vi "Encoder Angles.vi"(8 "Calibration Angle":dbl, 9 "Bottom Voltage":dbl, 10 "Top Voltage":dbl, 11 "AIDeviceRef Encoder":T1) -> (3 "Encoder Angle":dbl)   [LabVIEW 2013]
uses:
  <vilib>/Rock Robotics/WPI/AnalogChannel/WPI_AnalogChannelDevRef.ctl
  <vilib>/Rock Robotics/SystemInterfaces/Typedef/FPGA_TypedefAnalogModule.ctl
  <vilib>/Rock Robotics/SystemInterfaces/AI/FPGA_AIChannel.ctl
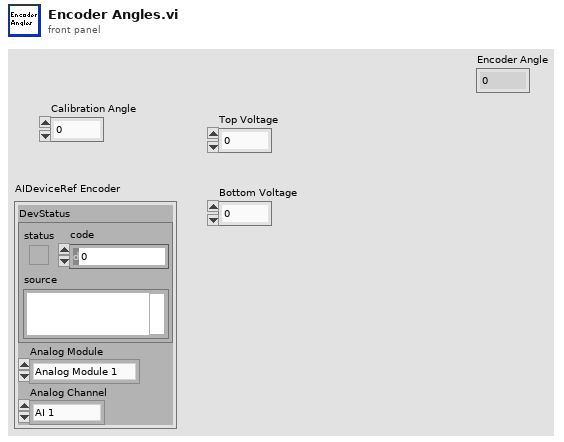
[diagram p1: front panel]
types:
  T1 = typedef "WPI_AnalogChannelDevRef.ctl" = cluster{"DevStatus":errorcluster, "Analog Module":T2, "Analog Channel":T3}
  T2 = typedef "FPGA_TypedefAnalogModule.ctl" = enum16{"Analog Module 1", "Analog Module 2"}
  T3 = typedef "FPGA_AIChannel.ctl" = enum8{"AI 1", "AI 2", "AI 3", "AI 4", "AI 5", "AI 6", "AI 7", "AI 8", "Invalid"}
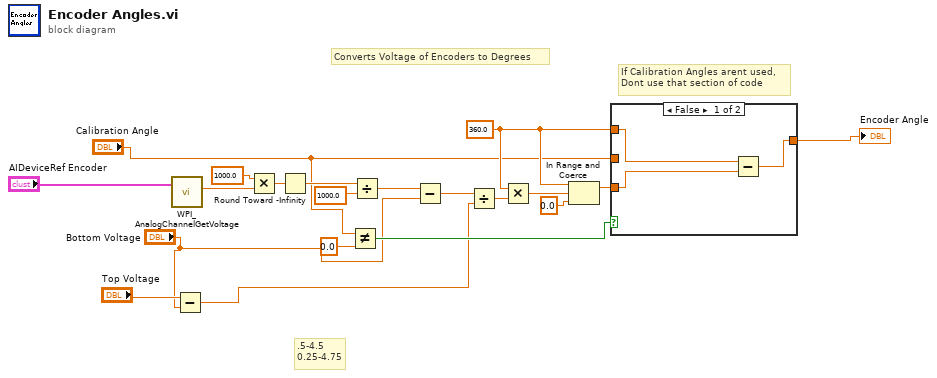
[diagram p0: block diagram]
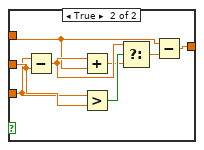
[diagram p2: hidden frame]
diagram:
  w10 = 360.0 ("y")
  # ".5-4.5\n0.25-4.75"
  # "Converts Voltage of Encoders to Degrees"
  # "If Calibration Angles arent used,\nDont use that section of code"
  n1 = call <vilib>:"WPI_AnalogChannelGetVoltage.vi"("AIDeviceRef"="AIDeviceRef Encoder") -> ("Voltage"=w16:dbl)  [unwired: 1 in, 9 out]
  n2 = Subtract(x="Top Voltage", y="Bottom Voltage") -> (x-y=w1:dbl)
  n3 = Multiply(x=1000.0 ("y"), y=w16) -> (x*y=w14:dbl)
  n4 = Round Toward -Infinity(1:w14) -> (0:w13:dbl)
  n5 = Not Equal?(x="Calibration Angle", y=0.0) -> (x != y?=w7:bool)
  n6 = Divide(x=w13, y=1000.0) -> (x/y=w11:dbl)
  n7 = Subtract(x=w11, y="Bottom Voltage") -> (x-y=w20:dbl)
  n8 = Divide(x=w20, y=w1) -> (x/y=w19:dbl)
  n9 = Multiply(x=w10, y=w19) -> (x*y=w18:dbl)
  n10 = In Range and Coerce(upper limit=w10, x=w18, lower limit=0.0) -> (coerced(x)=w9:dbl)  [unwired: 1 out]
  n11 = case shown="False" w7 {
    tunnel: w10 -> [w21 w27]
    tunnel: "Calibration Angle" -> [_ w26]
    tunnel: w9 -> [w22 w25]
    tunnel: [w23 w24] -> w8
    frame False {
      n12 = Subtract(x=w21, y=w22) -> (x-y=w23:dbl)
    }
    frame True {
      n13 = Subtract(x=w25, y=w26) -> (x-y=w30:dbl)
      n14 = Add(x=w30, y=w27) -> (x+y=w29:dbl)
      n15 = Greater?(x=w25, y=w26) -> (0:w31:bool)
      n16 = Select(t=w30, s=w31, f=w29) -> (s? t:f=w28:dbl)
      n17 = Subtract(x=w27, y=w28) -> (x-y=w24:dbl)
    }
  }
  "Encoder Angle" <- w8
